vi "ServoHostLatch.vi"(8 "error in":errorcluster, 9 "Enable":bool, 10 "Hi/Lo":bool, 11 "FPGA VI Reference In":T1) -> (0 "error out":errorcluster, 3 "FPGA VI Reference Out":T1)   [LabVIEW 2012]
uses:
  FPGA_ref.ctl
  <vilib>/Utility/error.llb/Error Cluster From Error Code.vi
  <vilib>/rvi/errors/niLvFpgaAdjustHostInterfaceError.vi
  <vilib>/rvi/interface/nirviReadWriteControl/nirviReadWriteControl.xnode
  NiFpgaLv.dll
  <vilib>/rvi/interface/Simulation/niFpgaSimulationCallBeginRW.vi
panel:
  out "pulse width (us)  2":i32
  in  "lower limit (Claw)":dbl=-1.0
  in  "upper limit (Claw)":dbl=1.0
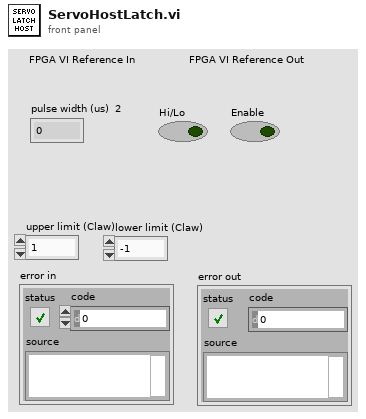
[diagram p1: front panel]
types:
  T1 = typedef "FPGA_ref.ctl" = refnum<k20>
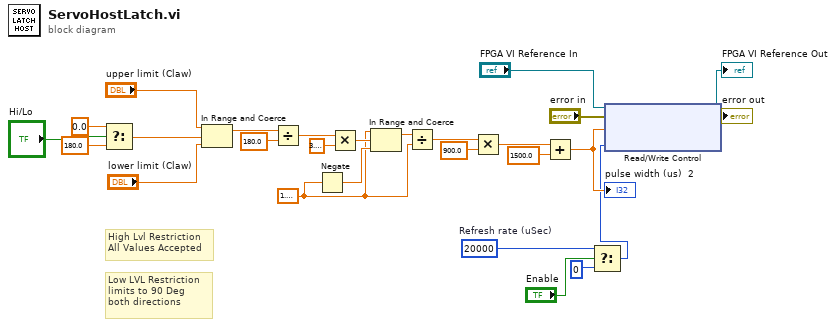
[diagram p0: block diagram]
diagram:
  w4 = u32 20000  # Refresh rate (uSec)
  w11 = 1.5707963267948966
  # "Low LVL Restriction\nlimits to 90 Deg \nboth directions"
  # "High Lvl Restriction\nAll Values Accepted"
  n1 = Select(t=0.0, s="Hi/Lo", f=180.0) -> (s? t:f=w8:dbl)
  n2 = In Range and Coerce(upper limit="upper limit (Claw)", x=w8, lower limit="lower limit (Claw)") -> (coerced(x)=w25:dbl)  [unwired: 1 out]
  n3 = Divide(x=w25, y=180.0) -> (x/y=w21:dbl)
  n4 = Negate(x=w11) -> (-x=w20:dbl)
  n5 = Multiply(x=w21, y=3.141592653589793) -> (x*y=w22:dbl)
  n6 = In Range and Coerce(upper limit=w11, x=w22, lower limit=w20) -> (coerced(x)=w12:dbl)  [unwired: 1 out]
  n7 = Divide(x=w12, y=w11) -> (x/y=w19:dbl)
  n8 = Multiply(x=w19, y=900.0) -> (x*y=w16:dbl)
  n9 = Add(x=w16, y=1500.0) -> (x+y=w13:dbl)
  "pulse width (us)  2" <- w13
  n10 = Select(t=w4, s="Enable", f=u32 0) -> (s? t:f=w1:u32)
  n11 = xnode "Read/Write Control"("FPGA VI Reference In"="FPGA VI Reference In", "error in"="error in", "servo Latch"=w13, "Count(uSec) Latch"=w1) -> ("FPGA VI Reference Out"=→"FPGA VI Reference Out":T1, "error out"=→"error out":errorcluster)
